vi "Rescript Msg.vi"() -> ()   [LabVIEW 2021]
uses:
  _Shared/_Shared.lvlib
  _Rescript Msg/_Rescript Msg/_Rescript Msg.lvclass
panel:
  in  "Rescript":bool
  in  "Name":string(combo)
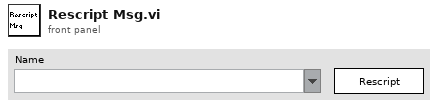
[diagram p1: front panel]
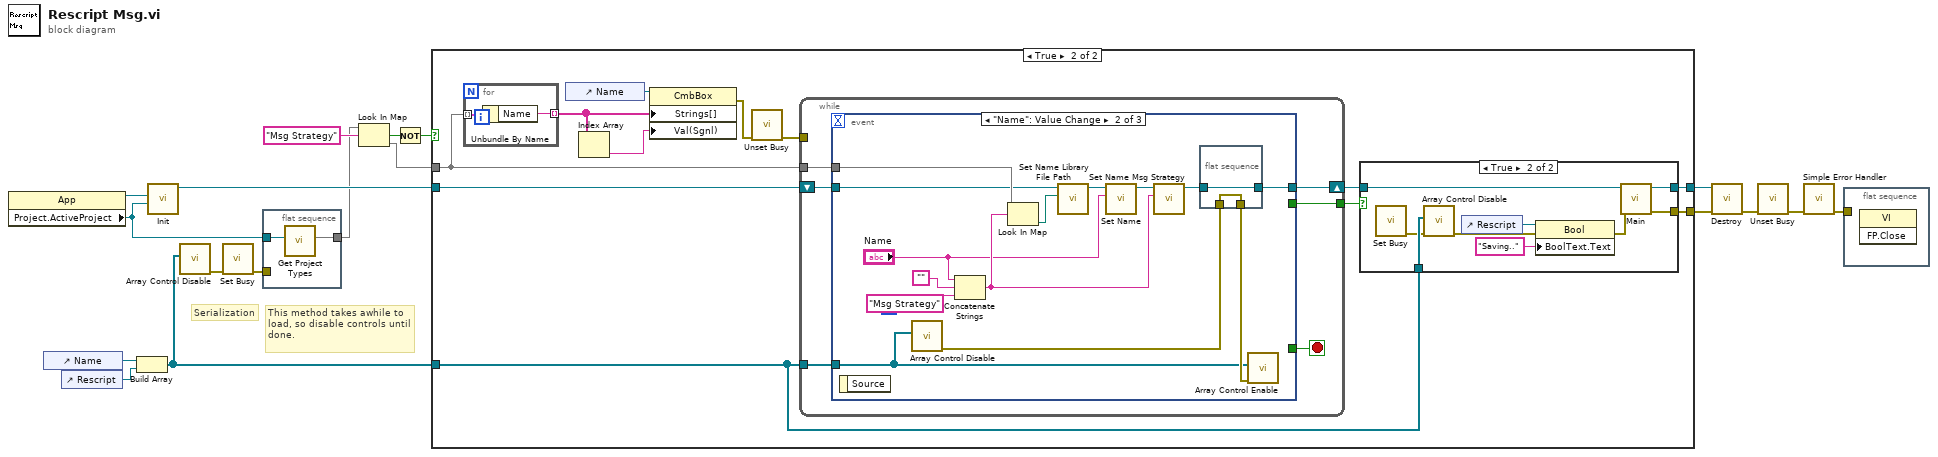
[diagram p0: block diagram]
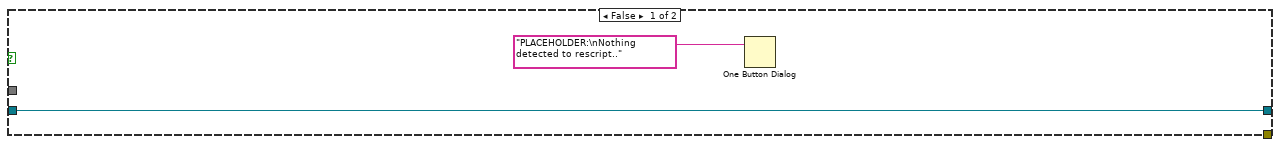
[diagram p2: hidden frame]
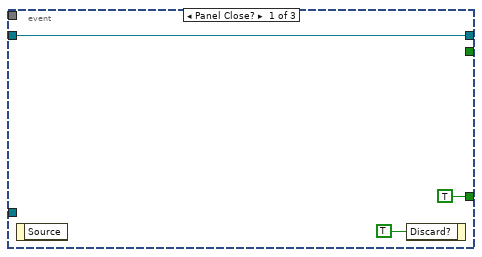
[diagram p4: hidden frame]
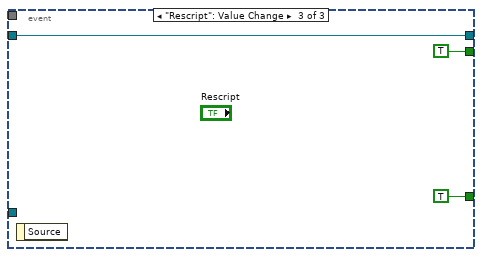
[diagram p5: hidden frame]
diagram:
  # "Serialization"
  # "This method takes awhile to load, so disable controls until done."
  n1 = property class="App"() -> (reference out=w13:refnum<vi>, "Project.ActiveProject"=w12:refnum<vi>)  [unwired: 2 in, 1 out]
  n2 = control-ref of="Name"() -> (w10:refnum<vi>)
  n3 = control-ref of="Rescript"() -> (w9:refnum<vi>)
  n4 = Build Array(w10, w9) -> (w18:refnum<vi>[])
  n5 = call "Init.vi"("Project:Active Project"=w12, "NI.LV.Dialog Instance"=w13) -> ("_Rescript Msg out"=w11:refnum<class "_Rescript Msg.lvclass">)  [unwired: 8 in, 1 out]
  n6 = call "Array Control Disable.vi"("Array Control in"=w18) -> ("error out"=w16:errorcluster)  [unwired: 10 in]
  n7 = call <vilib>:"Set Busy.vi"("error in (no error)"=w16) -> ("error out"=w15:errorcluster)  [unwired: 9 in, 1 out]
  n8 = flat-sequence {
    tunnel: w12 -> [w20]
    tunnel: [w19] -> w4
    tunnel: w15 -> [_]
    frame #0 {
      n9 = call "Get Project Types.vi"("Project:Active Project"=w20) -> ("Type Name Library File Path"=w19:map{string, map{string, path}})  [unwired: 10 in]
    }
  }
  n10 = Look In Map(map=w4, key="Msg Strategy" ("y")) -> (key not found?=w2:bool, value=w3:map{string, path})  [unwired: 1 in]
  n11 = Not(x=w2) -> (.not. x?=w1:bool)
  n12 = case shown="True" w1 {
    tunnel: w11 -> [w21 w31]
    tunnel: w3 -> [_ w25]
    tunnel: w18 -> [_ w29]
    tunnel: [w21 w30] -> w8
    tunnel: [_ w28] -> w7
    frame False {
      n13 = One Button Dialog(message="PLACEHOLDER:\nNothing detected to rescript..") -> ()  [unwired: 1 in, 1 out]
    }
    frame True {
      n14 = for {
        tunnel: w25 -> [w36] mode=indexing
        tunnel: [w35] -> w24 mode=indexing
        n15 = Unbundle By Name(w36) -> ("Name"=w35:string)
      }
      n16 = control-ref of="Name"() -> (w23:refnum<vi>)
      n17 = Index Array(array=w24) -> (element=w33:string)  [unwired: 1 in]
      n18 = property class="CmbBox"(reference=w23, "Strings[]"=w24, "Val(Sgnl)"=w33) -> (error out=w27:errorcluster)  [unwired: 1 in, 1 out]
      n19 = call <vilib>:"Unset Busy.vi"("error in (no error)"=w27) -> ("error out"=w26:errorcluster)  [unwired: 10 in]
      n20 = while {
        tunnel: [w52] -> w34
        tunnel: w26 -> [_]
        shift-right: [w49] -> w32
        shift-left: w31 -> [w50]
        tunnel: w25 -> [w48]
        tunnel: w29 -> [w47]
        stop <- w51 stop-if-true
        n21 = event shown="[1] \"Name\": Value Change" {
          selector: _ -> [_ _ _]
          dyn-events: _ -> [_ _ _]
          timeout: _ -> [_ _ _]
          tunnel: [_ _ TRUE ("Rename 2")] -> w52
          tunnel: [TRUE _ TRUE] -> w51
          tunnel: w50 -> [w53 w63 w74]
          tunnel: [w53 w67 w74] -> w49
          tunnel: w48 -> [_ w68 _]
          tunnel: w47 -> [_ w65 _]
          event Panel Close? {
            n22 = event-data() -> ()  [unwired: 1 in, 1 out]
            n23 = event-data("Discard?"=TRUE) -> ()  [unwired: 1 in, 1 out]
          }
          event "Name": Value Change {
            n24 = event-data() -> ()  [unwired: 1 in, 1 out]
            n25 = call "Array Control Disable.vi"("Array Control in"=w65) -> ("error out"=w66:errorcluster)  [unwired: 10 in]
            n26 = Concatenate Strings("Name", "", "Msg Strategy" ("string")) -> (w62:string)
            n27 = Look In Map(map=w68, key=w62) -> (value=w64:path)  [unwired: 1 in, 1 out]
            n28 = call "Set Name Library File Path.vi"("Name Library File Path"=w64, "_Rescript Msg in"=w63) -> ("_Rescript Msg out"=w59:refnum<class "_Rescript Msg.lvclass">)  [unwired: 9 in]
            n29 = call "Set Name.vi"("Name"="Name", "_Rescript Msg in"=w59) -> ("_Rescript Msg out"=w60:refnum<class "_Rescript Msg.lvclass">)  [unwired: 9 in]
            n30 = call "Set Name Msg Strategy.vi"("Name Msg Strategy"=w62, "_Rescript Msg in"=w60) -> ("_Rescript Msg out"=w58:refnum<class "_Rescript Msg.lvclass">)  [unwired: 9 in]
            n31 = flat-sequence {
              tunnel: [w71] -> w67
              tunnel: w58 -> [w71]
              tunnel: [w70] -> w69
              tunnel: w66 -> [w70]
              frame #0 {
              }
            }
            n32 = call "Array Control Enable.vi"("error in"=w69, "Array Control in"=w65) -> ()  [unwired: 9 in, 1 out]
          }
          event "Rescript": Value Change {
            n33 = event-data() -> ()  [unwired: 1 in, 1 out]
          }
        }
      }
      n34 = case shown="True" w34 {
        tunnel: w32 -> [w37 w42]
        tunnel: [w37 w41] -> w30
        tunnel: w29 -> [_ w44]
        tunnel: [_ w39] -> w28
        frame False {
        }
        frame True {
          n35 = call <vilib>:"Set Busy.vi"() -> ("error out"=w43:errorcluster)  [unwired: 10 in, 1 out]
          n36 = call "Array Control Disable.vi"("error in"=w43, "Array Control in"=w44) -> ("error out"=w46:errorcluster)  [unwired: 9 in]
          n37 = control-ref of="Rescript"() -> (w38:refnum<vi>)
          n38 = property class="Bool"(reference=w38, error in=w46, "BoolText.Text"="Saving.." ("Boolean Text.Text")) -> (error out=w40:errorcluster)  [unwired: 1 out]
          n39 = call "Main.vi"("error in"=w40, "_Rescript Msg in"=w42) -> ("error out"=w39:errorcluster, "_Rescript Msg out"=w41:refnum<class "_Rescript Msg.lvclass">)  [unwired: 8 in]
        }
      }
    }
  }
  n40 = call "Destroy.vi"("error in"=w7, "_Rescript Msg in"=w8) -> ("error out"=w6:errorcluster)  [unwired: 9 in]
  n41 = call <vilib>:"Unset Busy.vi"("error in (no error)"=w6) -> ("error out"=w14:errorcluster)  [unwired: 10 in]
  n42 = call <vilib>:"Simple Error Handler.vi"("error in (no error)"=w14) -> ("error out"=w17:errorcluster)  [unwired: 4 in, 4 out]
  n43 = flat-sequence {
    tunnel: w17 -> [_]
    frame #0 {
      n44 = invoke class="VI" method="FP.Close"() -> ()  [unwired: 3 in, 3 out]
    }
  }
